vi "add.data.to.buffer.vi"(8 "buffer.length":u8, 9 "buffer":u64[](array[numeric])=[0, 0, 0, 0, 0, 0, 0, 0, 0] format="%.0x", 11 "network Data Stream.ctl":cluster{"reset":bool, "Data Stream":T1} {"Data Stream"."data" format="%.0x"}) -> (2 "buffer.out":u64[](array[numeric]) format="%.0x", 3 "buffer.length.out":u8)   [LabVIEW 2020]
uses:
  <instrlib>/_niInstr/Network/Ethernet/Utility/v1/FPGA/Network Data Stream.ctl
  Market.Data.Common/fpga/fpganow.common.fpga.lvlib
  <instrlib>/_niInstr/Network/Ethernet/Utility/v1/FPGA/niInstr Ethernet Utilities FPGA v1.lvlib
panel:
  out "x rotated left by y":u64 format="%.0x"
  out "y":i8 format="%.0x"
  out "mask 2":u64 format="%.0x"
  out "mask":u64 format="%.0x"
  out "x .or. y?":u64 format="%.0x"
  out "old.value":u64 format="%.0x"
  out "new.value.u64":u64 format="%.0x"
  out "# of existing\nitems":u8
  out "Index":u8
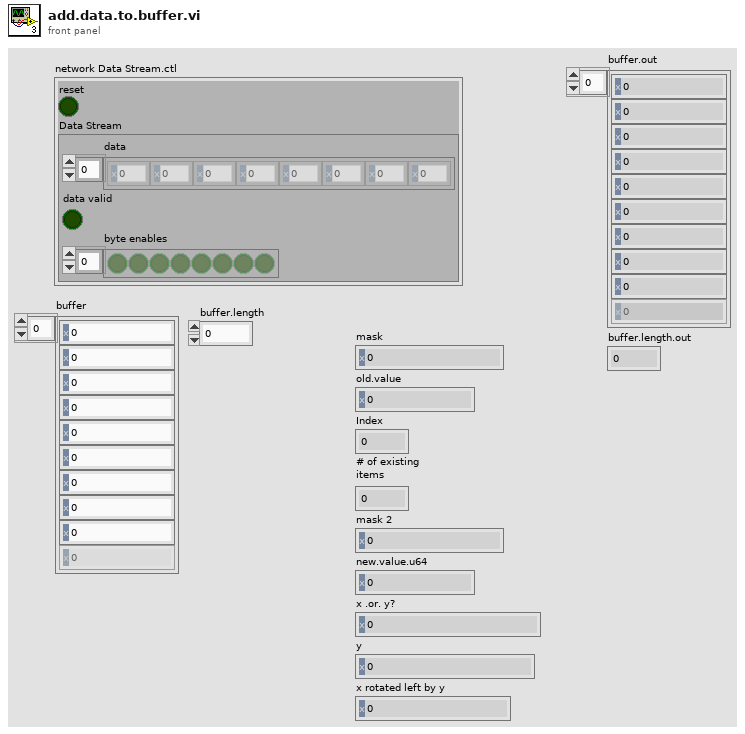
[diagram p1: front panel]
types:
  T1 = typedef "niInstr Ethernet Utilities FPGA v1.lvlib/Network Data Stream.ctl" = cluster{"data":u8[], "data valid":bool, "byte enables":bool[]}
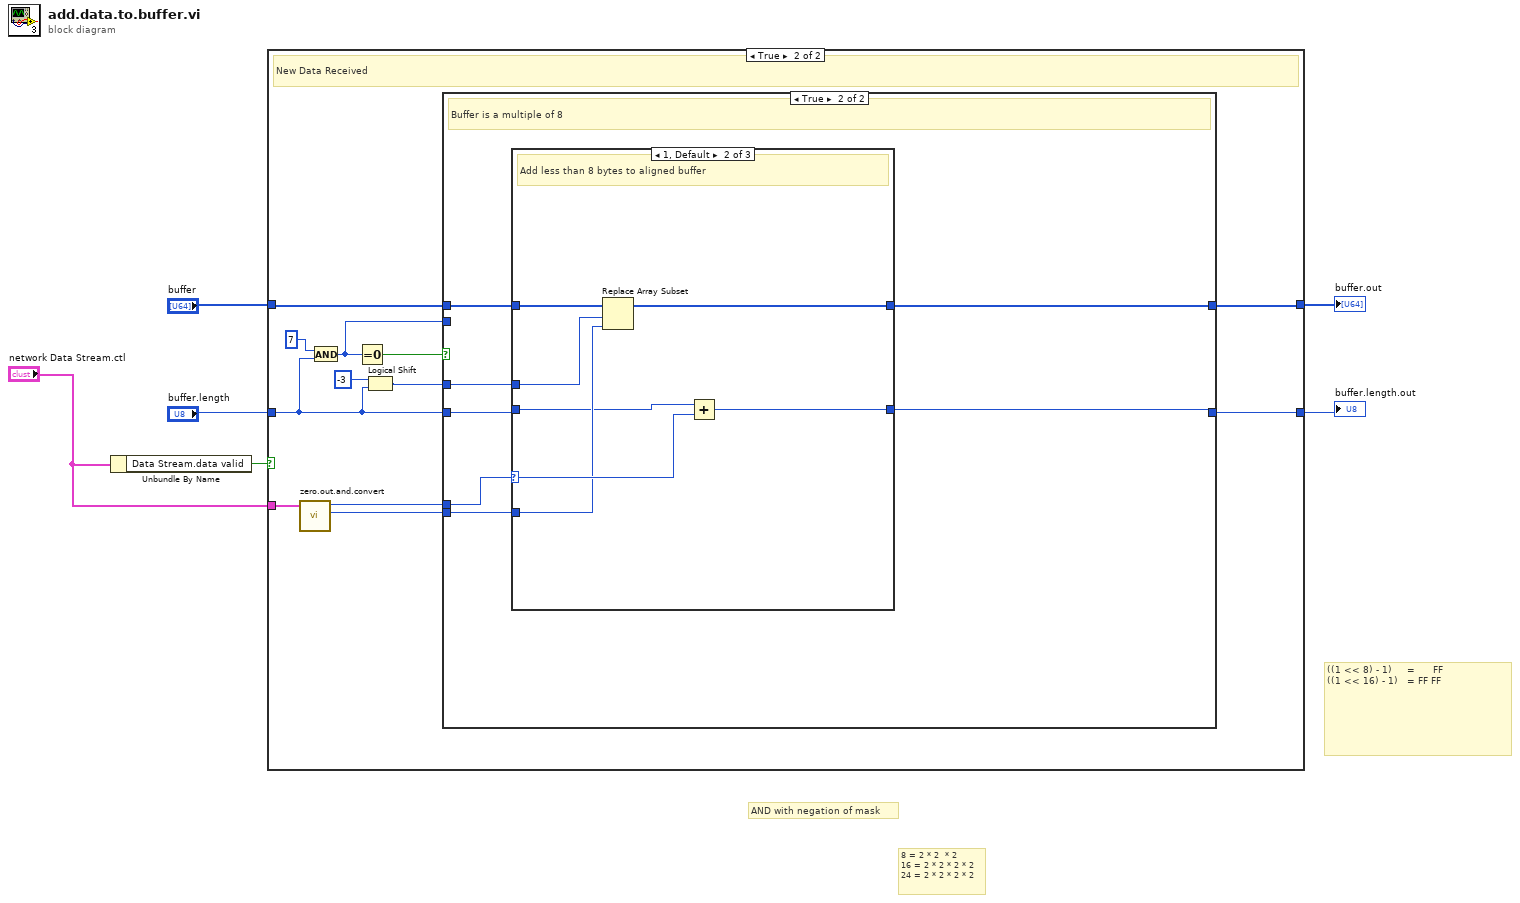
[diagram p0: block diagram]
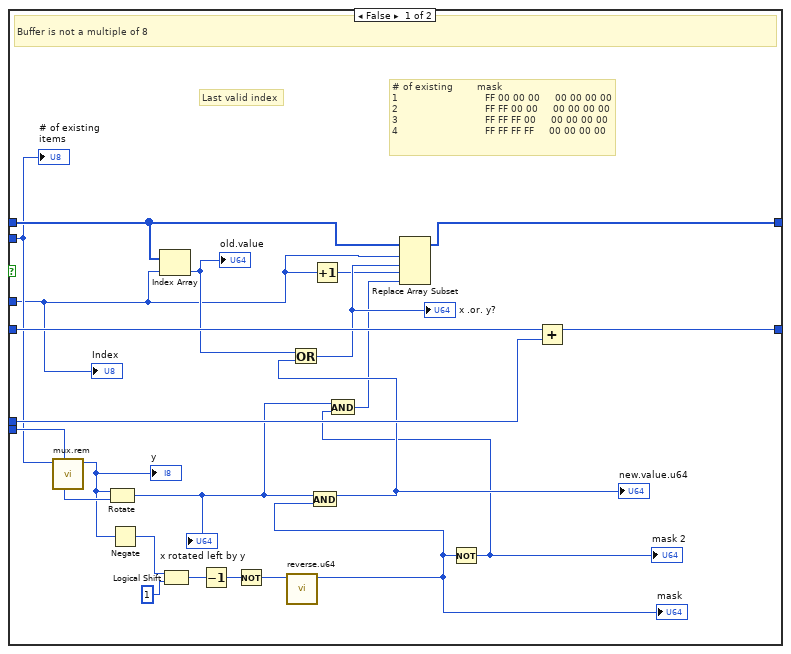
[diagram p3: hidden frame]
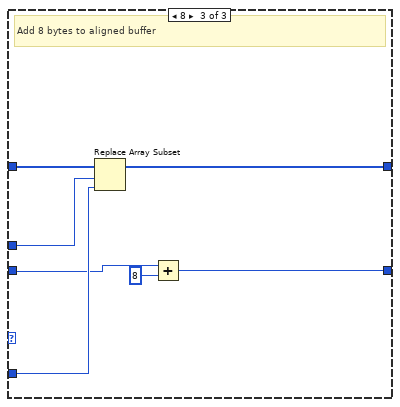
[diagram p5: hidden frame]
diagram:
  # "AND with negation of mask"
  # "8 = 2 * 2  * 2\n16 = 2 * 2 * 2 * 2\n24 = 2 * 2 * 2 * 2"
  # "((1 << 8) - 1)     =      FF\n((1 << 16) - 1)   = FF FF"
  n1 = Unbundle By Name("network Data Stream.ctl") -> ("Data Stream.data valid"=w2:bool)
  n2 = case shown="True" w2 {
    tunnel: "buffer.length" -> [w7 w15]
    tunnel: [w8 w19] -> w5
    tunnel: "buffer" -> [w8 w20]
    tunnel: [w7 w16] -> w3
    tunnel: "network Data Stream.ctl" -> [_ w9]
    frame False {
      # "Data is not valid - Noop"
    }
    frame True {
      # "New Data Received"
      n3 = call "zero.out.and.convert.vi"("network Data Stream.ctl"=w9) -> ("u64.be"=w11:u64, "Num.of.True"=w10:u8)  [unwired: 9 in]
      n4 = And(x=u8 7, y=w15) -> (x .and. y?=w12:u8)
      n5 = Equal To 0?(x=w12) -> (x = 0?=w17:bool)
      n6 = Logical Shift(y=i16 -3, x=w15) -> (x << y=w13:u8)
      n7 = case shown="True" w17 {
        tunnel: w20 -> [w41 w49]
        tunnel: [w39 w48] -> w19
        tunnel: w11 -> [w37 w47]
        tunnel: w10 -> [w35 w46]
        tunnel: w15 -> [w42 w45]
        tunnel: [w36 w44] -> w16
        tunnel: w13 -> [w26 w43]
        tunnel: w12 -> [w34 _]
        frame False {
          # "# of existing        mask\n1                             FF 00 00 00     00 00 00 00\n2                             FF FF 00 00     00 00 00 00\n3                             FF FF FF 00     00 00 00 00\n4                             FF FF FF FF     00 00 00 00"
          # "Last valid index"
          # "Buffer is not a multiple of 8"
          n8 = call "mux.rem.vi"("# of existing\nitems 3"=w34) -> ("y"=w31:i8)  [unwired: 10 in]
          "y" <- w31
          n9 = Rotate(1:w37, 2:w31) -> (0:w24:u64)
          "x rotated left by y" <- w24
          n10 = Negate(x=w31) -> (-x=w30:i8)
          n11 = Index Array(array=w41, index=w26) -> (element=w38:u64)
          "old.value" <- w38
          n12 = Logical Shift(y=w30, x=u64 1) -> (x << y=w33:u64)
          n13 = Decrement(x=w33) -> (x-1=w29:u64)
          n14 = Not(x=w29) -> (.not. x?=w28:u64)
          n15 = call "reverse.u64.vi"("U64.in"=w28) -> ("U64.reversed"=w21:u64)  [unwired: 10 in]
          "mask" <- w21
          n16 = And(x=w24, y=w21) -> (x .and. y?=w27:u64)
          "new.value.u64" <- w27
          n17 = Or(x=w38, y=w27) -> (x .or. y?=w40:u64)
          "x .or. y?" <- w40
          n18 = Increment(x=w26) -> (x+1=w25:u8)
          n19 = Not(x=w21) -> (.not. x?=w23:u64)
          "mask 2" <- w23
          n20 = And(x=w24, y=w23) -> (x .and. y?=w22:u64)
          n21 = Replace Array Subset(array=w41, new element #1=w40, index #1=w26, new element #2=w22, index #2=w25) -> (w39:u64[])
          n22 = Add(x=w42, y=w35) -> (x+y=w36:u8)
          "Index" <- w26
          "# of existing\nitems" <- w34
        }
        frame True {
          # "Buffer is a multiple of 8"
          n23 = case shown="1, Default" w46 {
            selector: w46 -> [_ w55 _]
            tunnel: w49 -> [w51 w58 w65]
            tunnel: w47 -> [_ w54 w64]
            tunnel: [w51 w57 w63] -> w48
            tunnel: [w50 w56 w61] -> w44
            tunnel: w45 -> [w50 w53 w62]
            tunnel: w43 -> [_ w52 w59]
            frame 0 {
              # "New new data - Noop"
            }
            frame 1, Default {
              # "Add less than 8 bytes to aligned buffer"
              n24 = Replace Array Subset(array=w58, new element=w54, index=w52) -> (w57:u64[])
              n25 = Add(x=w53, y=w55) -> (x+y=w56:u8)
            }
            frame 8 {
              # "Add 8 bytes to aligned buffer"
              n26 = Replace Array Subset(array=w65, new element=w64, index=w59) -> (w63:u64[])
              n27 = Add(x=w62, y=u8 8) -> (x+y=w61:u8)
            }
          }
        }
      }
    }
  }
  "buffer.out" <- w5
  "buffer.length.out" <- w3
